vi "indexEvent.vi"(8 "error in (no error)":errorcluster, 10 "ScriptEvent":refnum<class "ScriptEvent.lvclass">, 11 "ScriptEventList in":refnum<class "ScriptEventList.lvclass">) -> (0 "error out":errorcluster, 1 "eventId":dbl, 2 "ScriptEvent out":refnum<class "ScriptEvent.lvclass">, 3 "ScriptEventList out":refnum<class "ScriptEventList.lvclass">)   [LabVIEW 2009, in "Tools.lvlib" / "Scripting.lvlib" / "ScriptEventList.lvclass"]
uses:
  ScriptEventList.lvclass
  ScriptEvent.lvclass
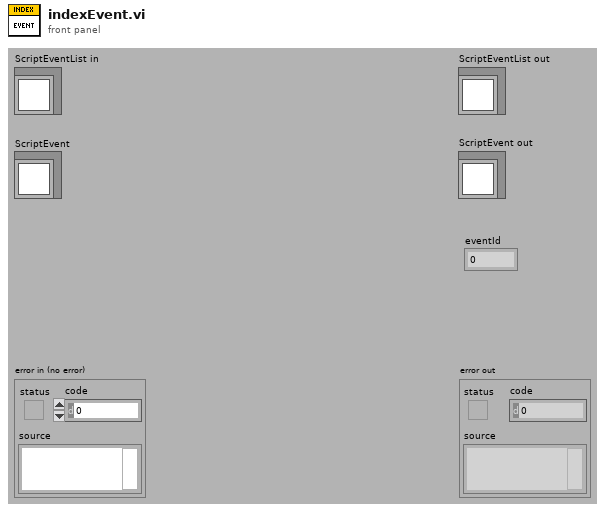
[diagram p1: front panel]
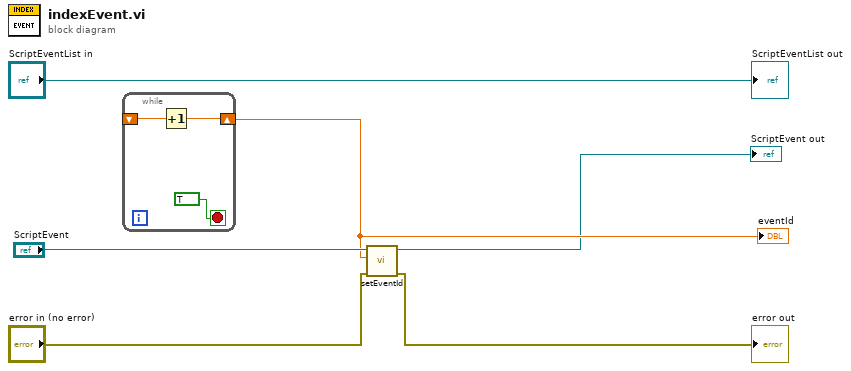
[diagram p0: block diagram]
diagram:
  n1 = while {
    shift-right: [w8] -> w2
    shift-left: _ -> [w7]
    stop <- TRUE stop-if-true
    n2 = Increment(x=w7) -> (x+1=w8:dbl)
  }
  "eventId" <- w2
  n3 = call-dynamic "setEventId.vi"("error in (no error)"="error in (no error)", "eventId"=w2, "ScriptEvent in"="ScriptEvent") -> ("error out"=→"error out":errorcluster, "ScriptEvent out"=→"ScriptEvent out":refnum<class "ScriptEvent.lvclass">)  [unwired: 7 in]
  "ScriptEventList out" <- "ScriptEventList in"
